vi "Parse LVClasses by Type.vi"(10 "Type":string, 11 "Input":string) -> (3 "Relative Paths":path[](array[path]))   [LabVIEW 2020, in "Test Finder.lvclass"]
uses:
  Test Finder.lvclass
  Test Finder.lvclass/Test Finder.ctl
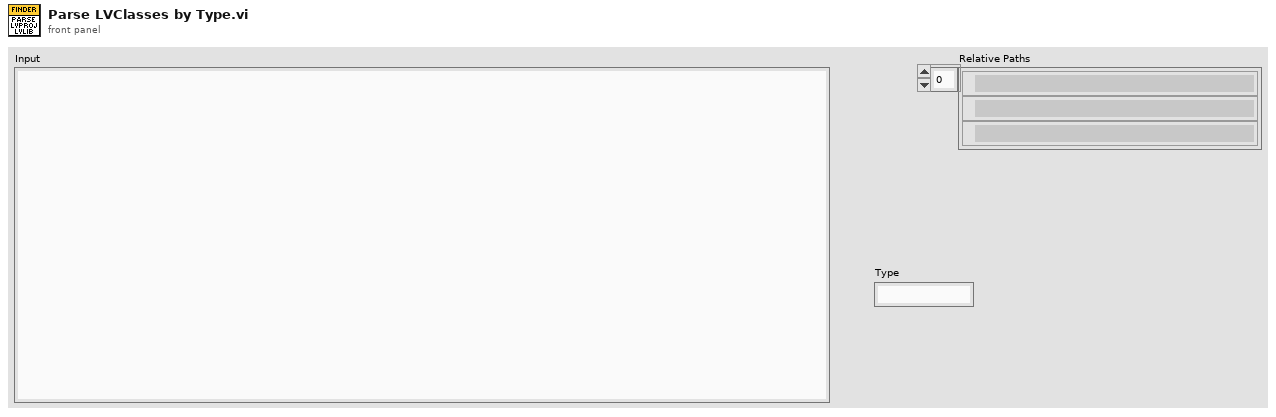
[diagram p1: front panel]
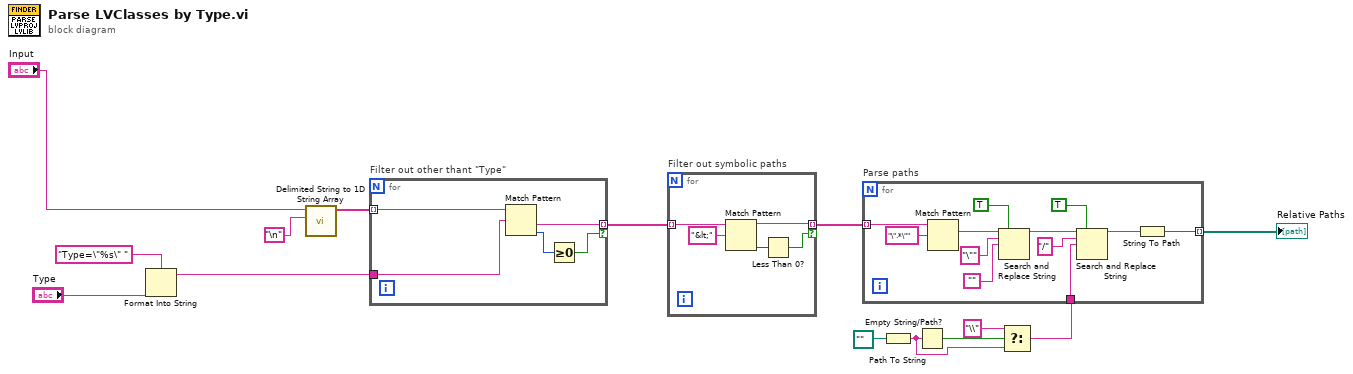
[diagram p0: block diagram]
diagram:
  n1 = Format Into String(format string="Type=\"%s\" " ("regular expression"), "Type") -> (resulting string=w9:string)  [unwired: 2 in, 1 out]
  n2 = call <vilib>:"Delimited String to 1D String Array.vi"("delimiter"="\n", "delimited string"="Input") -> ("string array"=w13:string[])  [unwired: 9 in]
  n3 = for "Filter out other thant \"Type\"" {
    tunnel: w13 -> [w19] mode=indexing
    tunnel: [w18] -> w6 mode=indexing if=w16
    tunnel: w9 -> [w15]
    n4 = Match Pattern(string=w19, regular expression=w15) -> (after substring=w18:string, offset past match=w17:i32)  [unwired: 1 in, 2 out]
    n5 = Greater Or Equal To 0?(x=w17) -> (x >= 0?=w16:bool)
  }
  n6 = for "Filter out symbolic paths" {
    tunnel: [w23] -> w7 mode=indexing if=w20
    tunnel: w6 -> [w24] mode=indexing
    n7 = Match Pattern(string=w24, regular expression="&lt;") -> (before substring=w23:string, offset past match=w21:i32)  [unwired: 1 in, 2 out]
    n8 = Less Than 0?(x=w21) -> (x < 0?=w20:bool)
  }
  n9 = Path To String(path=path "") -> (string=w1:string)
  n10 = Empty String/Path?(string/path=w1) -> (empty?=w3:bool)
  n11 = Select(t="\\" ("search string"), s=w3, f=w1) -> (s? t:f=w5:string)
  n12 = for "Parse paths" {
    tunnel: w7 -> [w36] mode=indexing
    tunnel: [w29] -> w8 mode=indexing
    tunnel: w5 -> [w25]
    n13 = Match Pattern(string=w36, regular expression="\".*\"") -> (match substring=w34:string)  [unwired: 1 in, 3 out]
    n14 = Search and Replace String(replace all?=TRUE ("replace all? (F)"), input string=w34, search string="\"", replace string="") -> (result string=w30:string)  [unwired: 4 in, 3 out]
    n15 = Search and Replace String(replace all?=TRUE ("replace all? (F)"), input string=w30, search string="/", replace string=w25) -> (result string=w28:string)  [unwired: 4 in, 3 out]
    n16 = String To Path(string=w28) -> (path=w29:path)
  }
  "Relative Paths" <- w8
